vi "To Text-Complete.vi"(6 "selected path":path, 7 "Header":string, 8 "error in (no error)":errorcluster, 10 "PTP Array":dbl[](array[numeric]), 11 "SGP Array":dbl[](array[numeric])) -> (0 "error out":errorcluster, 2 "resulting string":string)   [LabVIEW 2013]
panel:
  out "Trial":string
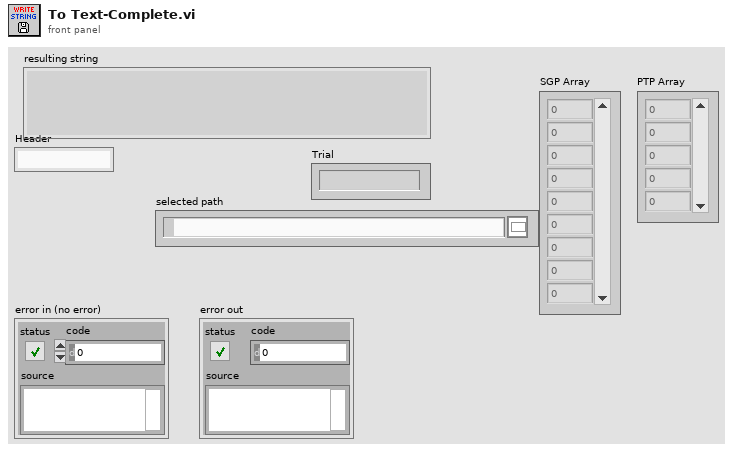
[diagram p1: front panel]
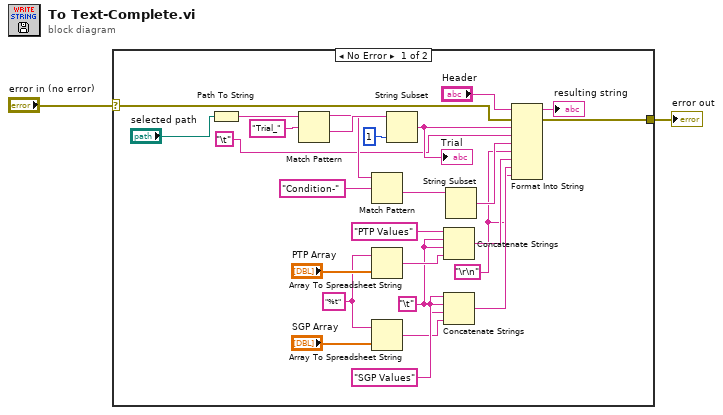
[diagram p0: block diagram]
diagram:
  n1 = case shown="No Error" "error in (no error)" {
    selector: "error in (no error)" -> [w26 w29]
    tunnel: [w25 w29] -> w1
    frame No Error {
      w3 = "\t"
      w17 = "%t" ("format string")
      w6 = "\r\n"
      n2 = Path To String(path="selected path") -> (string=w14:string)
      n3 = Match Pattern(string=w14, regular expression="Trial_") -> (before substring=w13:string, after substring=w23:string)  [unwired: 1 in, 2 out]
      n4 = Match Pattern(string=w13, regular expression="Condition-") -> (after substring=w12:string)  [unwired: 1 in, 3 out]
      n5 = Array To Spreadsheet String(array="PTP Array", 3:w17) -> (spreadsheet string=w4:string)  [unwired: 1 in]
      n6 = Array To Spreadsheet String(array="SGP Array", 3:w17) -> (spreadsheet string=w5:string)  [unwired: 1 in]
      n7 = String Subset(string=w23, length (rest)=1 ("length (rest)")) -> (substring=w20:string)  [unwired: 1 in]
      "Trial" <- w20
      n8 = Concatenate Strings("PTP Values" ("string"), w3, w3, w4) -> (w10:string)
      n9 = Concatenate Strings("SGP Values" ("string"), w3, w3, w5) -> (w7:string)
      n10 = String Subset(string=w12) -> (substring=w11:string)  [unwired: 2 in]
      n11 = Format Into String(initial string="Header", error in=w26, w20, "\t", w11, w6, w10, w7, w6) -> (resulting string=→"resulting string":string, error out=w25:errorcluster)  [unwired: 1 in]
    }
    frame Error {
    }
  }
  "error out" <- w1
